vi "ParseInputs.vi"(8 "error in (no error)":errorcluster, 10 "Inputs":string[](array[string]), 11 "RunTests in":refnum<class "RunVITester.lvclass">) -> (0 "error out":errorcluster, 3 "RunTests out":refnum<class "RunVITester.lvclass">)   [LabVIEW 2015, in "RunVITester.lvclass"]
uses:
  RunVITester.lvclass
  RunVITester.lvclass/RunVITester.ctl
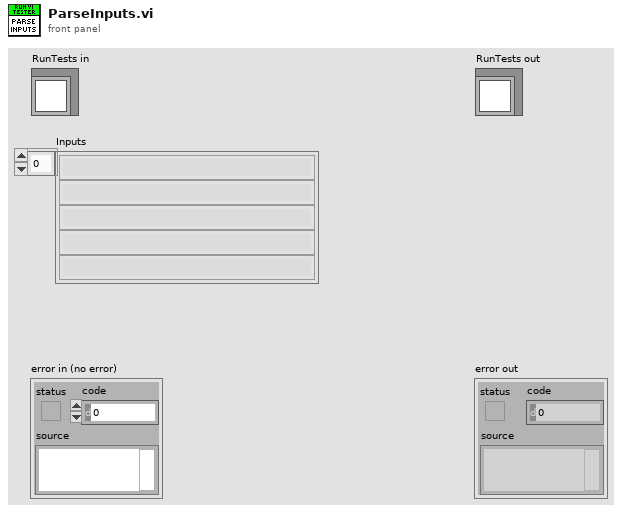
[diagram p1: front panel]
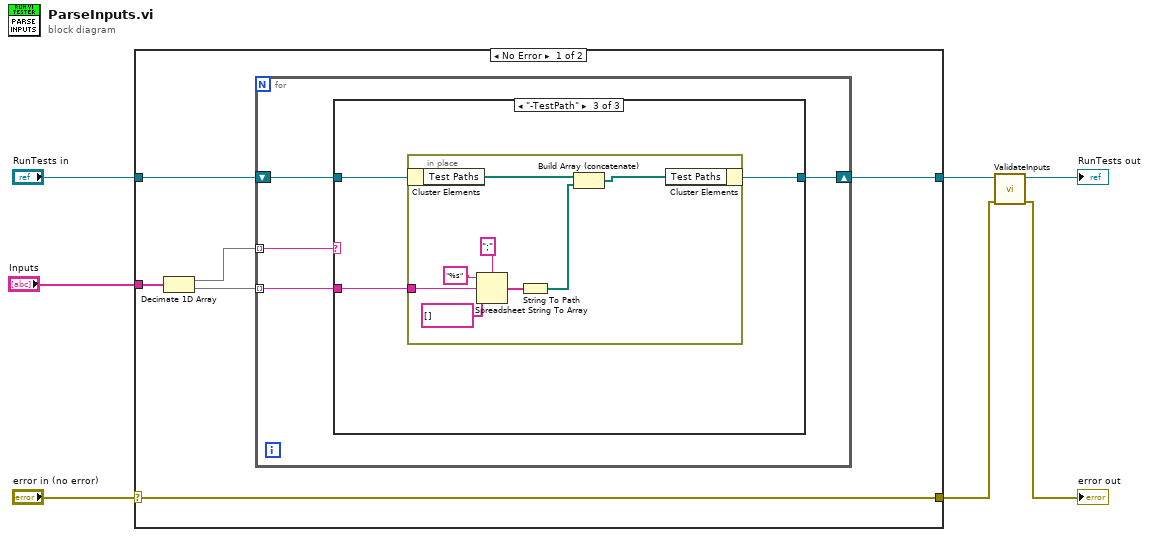
[diagram p0: block diagram]
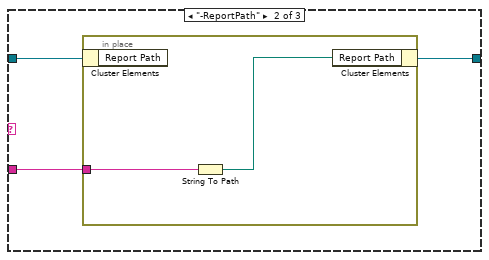
[diagram p3: hidden frame]
diagram:
  n1 = case shown="No Error" "error in (no error)" {
    selector: "error in (no error)" -> [w13 w36]
    tunnel: [w13 w36] -> w2
    tunnel: [w10 w35] -> w4
    tunnel: "RunTests in" -> [w11 w35]
    tunnel: "Inputs" -> [w12 _]
    frame No Error {
      n2 = Decimate 1D Array(w12) -> (w9:string[], w8:string[])
      n3 = for {
        shift-right: [w14] -> w10
        shift-left: w11 -> [w15]
        tunnel: w9 -> [w17] mode=indexing
        tunnel: w8 -> [w16] mode=indexing
        n4 = case shown="\"-TestPath\"" w17 {
          tunnel: w16 -> [_ w20 w25]
          tunnel: w15 -> [w18 w21 w26]
          tunnel: [w18 w19 w24] -> w14
          frame Default {
          }
          frame "-ReportPath" {
            n5 = in-place {
              in-place-border: w20 -> [w23]
              n6 = in-place-cluster #1(w21) -> ()  [unwired: 1 out]
              n7 = String To Path(string=w23) -> (path=w22:path)
              n8 = in-place-cluster #1("Report Path"=w22) -> (w19:refnum<class "RunVITester.lvclass">)
            }
          }
          frame "-TestPath" {
            n9 = in-place {
              in-place-border: w25 -> [w30]
              n10 = in-place-cluster #2(w26) -> ("Test Paths"=w34:path[])
              n11 = Spreadsheet String To Array(delimiter (Tab)=";", format string="%s", spreadsheet string=w30, array type (2D Dbl)=string[] []) -> (array=w29:string[])
              n12 = String To Path(string=w29) -> (path=w32:path[])
              n13 = Build Array (concatenate)(w34, w32) -> (w33:path[])
              n14 = in-place-cluster #2("Test Paths"=w33) -> (w24:refnum<class "RunVITester.lvclass">)
            }
          }
        }
      }
    }
    frame Error {
    }
  }
  n15 = call "ValidateInputs.vi"("error in (no error)"=w2, "RunTests in"=w4) -> ("error out"=→"error out":errorcluster, "RunTests out"=→"RunTests out":refnum<class "RunVITester.lvclass">)  [unwired: 8 in]
